vi "toDevVarLongStringArray.vi"(1 "ArgIO":cluster{"num data":u8[], "str data":string[]}) -> (0 "argout":cluster{"lvalue":i32[], "svalue":string[]})   [LabVIEW 2014, in "tango.lvlib"]
uses:
  tango.lvlib
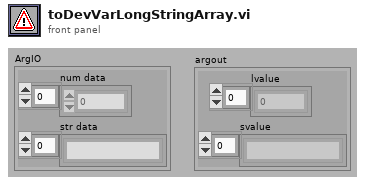
[diagram p1: front panel]
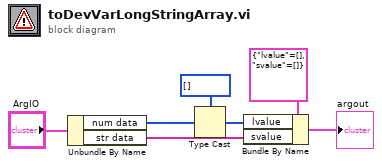
[diagram p0: block diagram]
diagram:
  n1 = Unbundle By Name("ArgIO") -> ("num data"=w5:u8[], "str data"=w1:string[])
  n2 = Type Cast(type=i32[] [], x=w5) -> (*(type *) &x=w4:i32[])
  n3 = Bundle By Name(cluster=cluster{"lvalue":i32[], "svalue":string[]} {"lvalue"=[], "svalue"=[]} ("argin"), "lvalue"=w4, "svalue"=w1) -> (→"argout":cluster{"lvalue":i32[], "svalue":string[]})
